vi "S_ReadProperty.vi"(8 "error in (no error)":errorcluster, 11 "reference in":refnum<class "SubTemplate.lvclass">) -> (0 "error out":errorcluster, 2 "property":dbl, 3 "reference out":refnum<class "SubTemplate.lvclass">)   [LabVIEW 2020]
uses:
  <resource>/Framework/Providers/Open_GDS/ClassProviders/Provider_EndevoGOOP300/Templates/SubTemplate/SubTemplate.lvclass
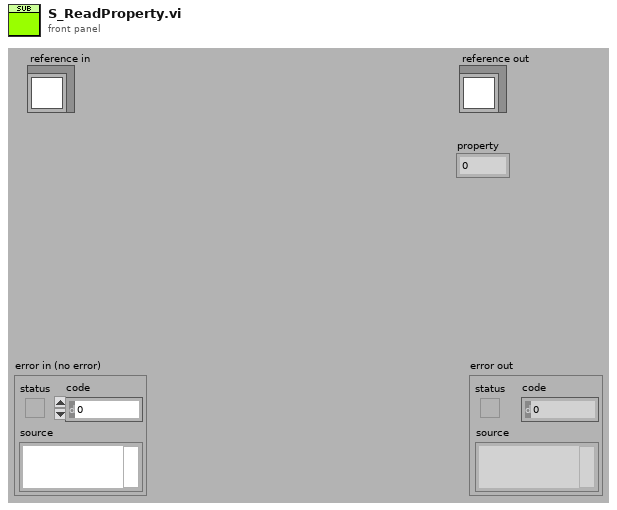
[diagram p1: front panel]
types:
  T1 = typedef "SubTemplate.lvclass/ObjectAttributes.ctl" = cluster{"Base class":T2}
  T2 = typedef "BaseTemplate.lvclass/ObjectAttributes.ctl" = cluster{"Attribute1":dbl}
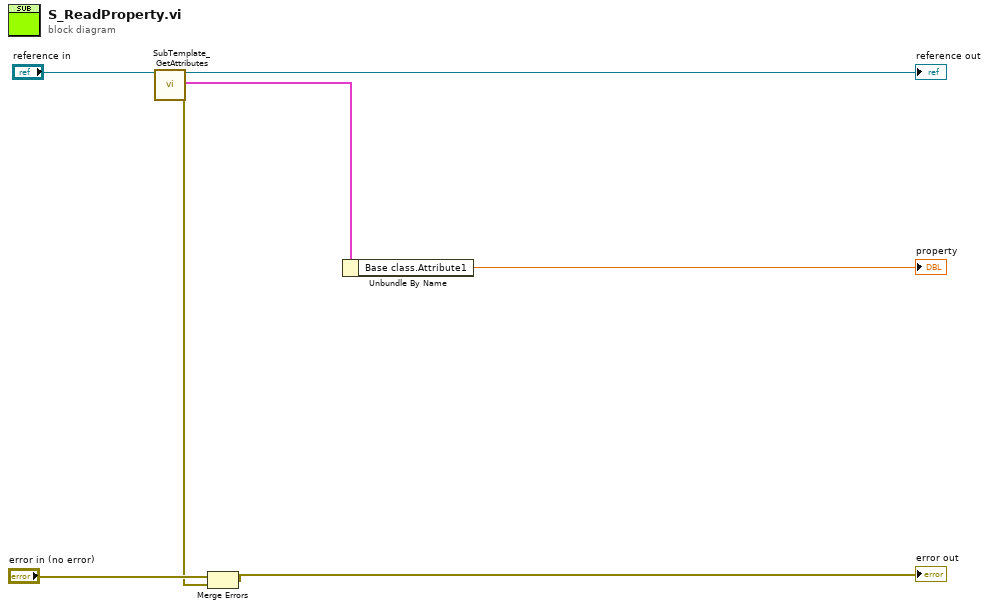
[diagram p0: block diagram]
diagram:
  n1 = call <resource>:"SubTemplate_GetAttributes.vi"("reference in"="reference in") -> ("reference out"=→"reference out":refnum<class "SubTemplate.lvclass">, "Attributes"=w4:T1, "error out"=w2:errorcluster)  [unwired: 15 in, 1 out]
  n2 = Merge Errors("error in (no error)", w2) -> (→"error out":errorcluster)
  n3 = Unbundle By Name(w4) -> ("Base class.Attribute1"=→"property":dbl)
